vi "ManualHoodControl.vi"(6 "Down":bool, 7 "Up":bool, 8 "Top":T1, 9 "AIDeviceRef":T4, 11 "Bottom":T1) -> (0 "Hood Speed":dbl, 1 "Voltage":dbl, 2 "Shoter Angle":dbl)   [LabVIEW 2011]
uses:
  <vilib>/Rock Robotics/WPI/AnalogChannel/WPI_AnalogChannelDevRef.ctl
  <vilib>/Rock Robotics/SystemInterfaces/Typedef/FPGA_TypedefAnalogModule.ctl
  <vilib>/Rock Robotics/SystemInterfaces/AI/FPGA_AIChannel.ctl
  <vilib>/Rock Robotics/WPI/DigitalInput/WPI_DigitalInputDevRef.ctl
  <vilib>/Rock Robotics/SystemInterfaces/DIO/FPGA_DIOChannel.ctl
  <vilib>/Rock Robotics/SystemInterfaces/Typedef/FPGA_TypedefDigitalModule.ctl
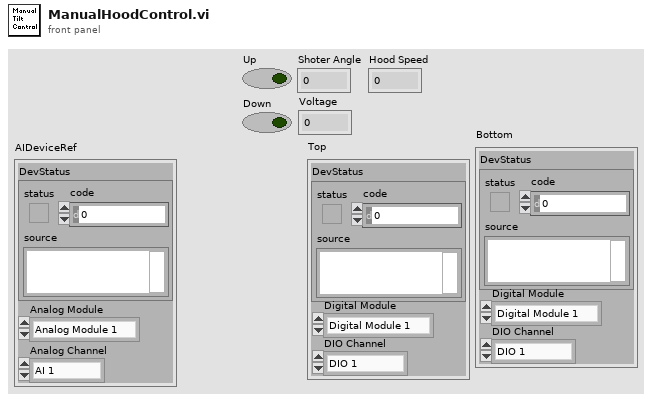
[diagram p1: front panel]
types:
  T1 = typedef "WPI_DigitalInputDevRef.ctl" = cluster{"DevStatus":errorcluster, "DIO Channel":T2, "Digital Module":T3}
  T2 = typedef "FPGA_DIOChannel.ctl" = enum8{"DIO 1", "DIO 2", "DIO 3", "DIO 4", "DIO 5", "DIO 6", "DIO 7", "DIO 8", "DIO 9", "DIO 10", "DIO 11", "DIO 12", "DIO 13", "DIO 14", "Invalid"}
  T3 = typedef "FPGA_TypedefDigitalModule.ctl" = enum16{"Digital Module 1", "Digital Module 2"}
  T4 = typedef "WPI_AnalogChannelDevRef.ctl" = cluster{"DevStatus":errorcluster, "Analog Module":T5, "Analog Channel":T6}
  T5 = typedef "FPGA_TypedefAnalogModule.ctl" = enum16{"Analog Module 1", "Analog Module 2"}
  T6 = typedef "FPGA_AIChannel.ctl" = enum8{"AI 1", "AI 2", "AI 3", "AI 4", "AI 5", "AI 6", "AI 7", "AI 8", "Invalid"}
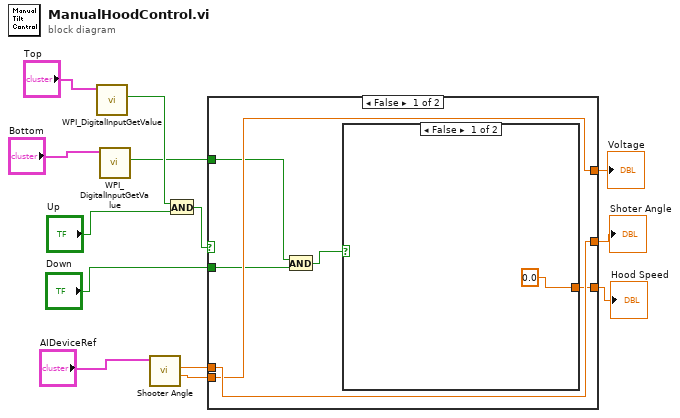
[diagram p0: block diagram]
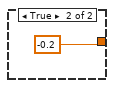
[diagram p2: hidden frame]
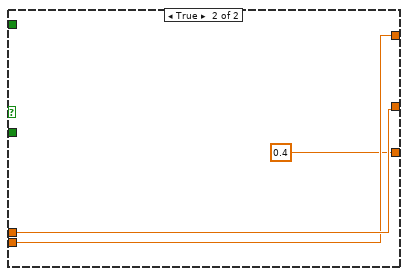
[diagram p3: hidden frame]
diagram:
  n1 = call <vilib>:"WPI_DigitalInputGetValue.vi"("DigitalInputDevRef"="Top") -> ("Value"=w4:bool)  [unwired: 8 in, 2 out]
  n2 = call <vilib>:"WPI_DigitalInputGetValue.vi"("DigitalInputDevRef"="Bottom") -> ("Value"=w2:bool)  [unwired: 8 in, 2 out]
  n3 = call "Shooter Angle.vi"("AIDeviceRef"="AIDeviceRef") -> ("Voltage"=w8:dbl, "Shoter Angle"=w9:dbl)  [unwired: 9 in]
  n4 = And(x=w4, y="Up") -> (x .and. y?=w12:bool)
  n5 = case shown="False" w12 {
    tunnel: [w19 w24] -> w10
    tunnel: w9 -> [w19 w24]
    tunnel: [w18 w23] -> w7
    tunnel: w8 -> [w18 w23]
    tunnel: "Down" -> [w16 _]
    tunnel: w2 -> [w15 _]
    tunnel: [w14 0.4 ("Hood Speed")] -> w1
    frame False {
      n6 = And(x=w15, y=w16) -> (x .and. y?=w17:bool)
      n7 = case shown="False" w17 {
        tunnel: [0.0 ("Hood Speed") -0.2 ("Hood Speed")] -> w14
        frame False {
        }
        frame True {
        }
      }
    }
    frame True {
    }
  }
  "Shoter Angle" <- w10
  "Voltage" <- w7
  "Hood Speed" <- w1
